vi "PCO_Bayer.vi"() -> (0 "PCO_Bayer":cluster{"iKernel":i32, "iColorMode":i32} {"iKernel" items=["BAYER_UPPER_LEFT_IS_RED", "BAYER_UPPER_LEFT_IS_GREEN_RED", "BAYER_UPPER_LEFT_IS_GREEN_BLUE", "BAYER_UPPER_LEFT_IS_BLUE"]}, 1 "PCO_Bayer_Raw":T1, 2 "Length":u16, 3 "Raw_Length":u16)   [LabVIEW 2019, in "Convert.lvlib"]
doc: "Use this template to build a VI to use as a subVI."
uses:
  Convert.lvlib
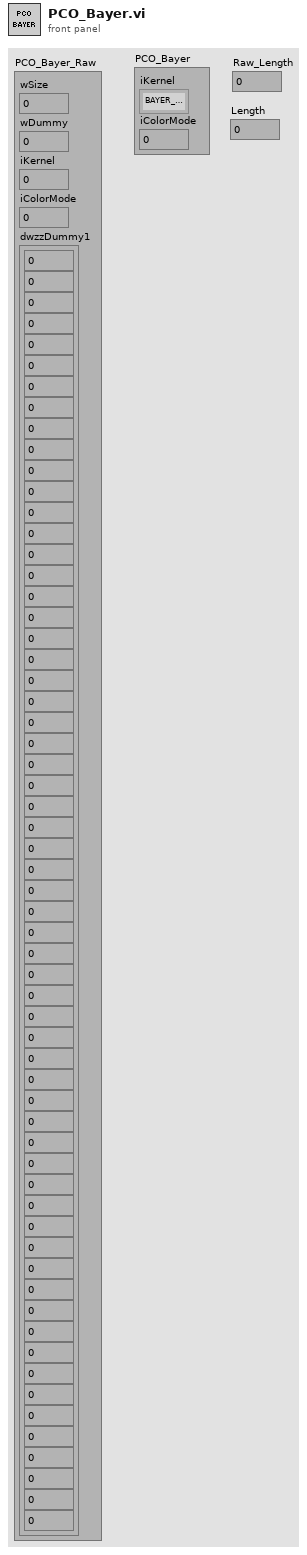
[diagram p1: front panel]
types:
  T1 = cluster{"wSize":u16, "wDummy":u16, "iKernel":i32, "iColorMode":i32, "dwzzDummy1":cluster{u32, u32, u32, u32, u32, u32, u32, u32, u32, u32, u32, u32, u32, u32, u32, u32, u32, u32, u32, u32, u32, u32, u32, u32, u32, u32, u32, u32, u32, u32, u32, u32, u32, u32, u32, u32, u32, u32, u32, u32, u32, u32, u32, u32, u32, u32, u32, u32, u32, u32, u32, u32, u32, u32, u32, u32, u32, u32, u32, u32, u32}}
  T2 = cluster{u32, u32, u32, u32, u32, u32, u32, u32, u32, u32, u32, u32, u32, u32, u32, u32, u32, u32, u32, u32, u32, u32, u32, u32, u32, u32, u32, u32, u32, u32, u32, u32, u32, u32, u32, u32, u32, u32, u32, u32, u32, u32, u32, u32, u32, u32, u32, u32, u32, u32, u32, u32, u32, u32, u32, u32, u32, u32, u32, u32, u32}
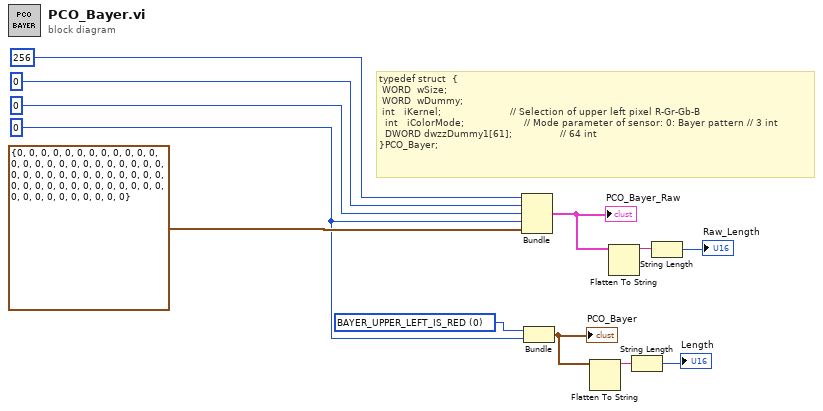
[diagram p0: block diagram]
diagram:
  w1 = 0 items=["BAYER_UPPER_LEFT_IS_RED", "BAYER_UPPER_LEFT_IS_GREEN_RED", "BAYER_UPPER_LEFT_IS_GREEN_BLUE", "BAYER_UPPER_LEFT_IS_BLUE"] ("iKernel")
  w2 = 0 ("iColorMode")
  # "typedef struct  {\n\tWORD  wSize;\n\tWORD  wDummy;\n\tint   iKernel;                       // Selection of upper left pixel R-Gr-Gb-B\n  int   iColorMode;                    // Mode parameter of sensor: 0: Bayer pattern // 3 int\n  DWORD dwzzDummy1[61];                // 64 int\n}PCO_Bayer;"
  n1 = Bundle("wSize"=u16 256, "wDummy"=u16 0, "iKernel"=0, "iColorMode"=w2, "dwzzDummy1"=T2 {0, 0, 0, 0, 0, 0, 0, 0, 0, 0, 0, 0, 0, 0, 0, 0, 0, 0, 0, 0, 0, 0, 0, 0, 0, 0, 0, 0, 0, 0, 0, 0, 0, 0, 0, 0, 0, 0, 0, 0, 0, 0, 0, 0, 0, 0, 0, 0, 0, 0, 0, 0, 0, 0, 0, 0, 0, 0, 0, 0, 0}) -> (w6:T1)  [unwired: 1 in]
  "PCO_Bayer_Raw" <- w6
  n2 = Bundle("iKernel"=w1, "iColorMode"=w2) -> (w12:cluster{"iKernel":i32, "iColorMode":i32})  [unwired: 1 in]
  "PCO_Bayer" <- w12
  n3 = Flatten To String(anything=w12) -> (data string=w11:string)  [unwired: 3 in, 2 out]
  n4 = Flatten To String(anything=w6) -> (data string=w10:string)  [unwired: 3 in, 2 out]
  n5 = String Length(string=w11) -> (length=→"Length":i32)
  n6 = String Length(string=w10) -> (length=→"Raw_Length":i32)
